vi "CRYSelect Massages.vi"(0 "Data in":T3 {"Z data" items=["dB", "Lin"]; "X data" items=["dB", "Lin"]; "Y data" items=["dB", "Lin"]; "Z dB ref" format="%.1f"; "Z axis" items=["Log", "Lin"]; "X dB ref" format="%.1f"; "X axis" items=["Log", "Lin"]; "Y axis" items=["Log", "Lin"]; "Y dB ref" format="%.1f"; "Curve"."z" format="%.2f"; "Curve"."y" format="%.2f"; "Curve"."x" format="%.2f"}, 5 "Results in":T1 {"Margin" format="%.2f"}, 7 "Mode":u16(slide), 9 "Dat_State":bool[](array[boolean]), 11 "Res_state":bool[](array[boolean]), 12 "USL":dbl, 13 "LSL":dbl) -> (4 "Run flag":bool)   [LabVIEW 2013]
uses:
  Typedef Control/CRYData Cluster Array.ctl
  Typedef Control/CRYData Cluster.ctl
  Typedef Control/CRYResult Cluster Array.ctl
  Typedef Control/CRYResult Cluster.ctl
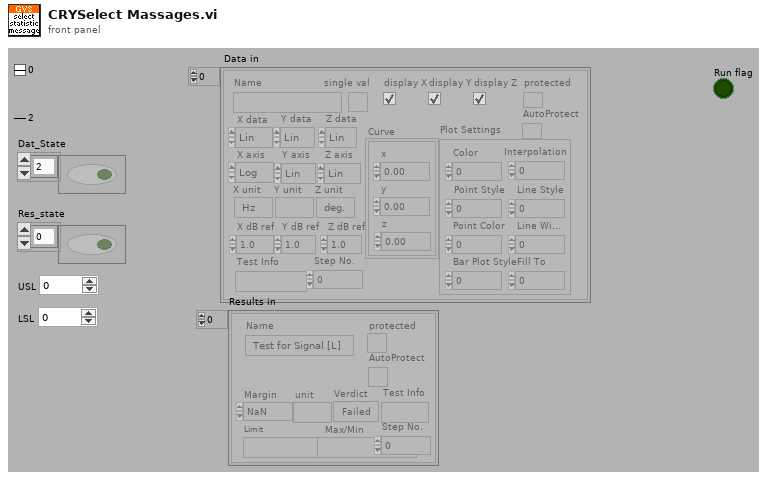
[diagram p1: front panel]
types:
  T1 = typedef "CRYResult Cluster Array.ctl" = T2[]
  T2 = typedef "CRYResult Cluster.ctl" = cluster{"Name":string, "Margin":dbl, "unit":string, "Verdict":bool, "Limit":string, "Max/Min":string, "protected":bool, "Step No.":i32, "Test Info":string, "AutoProtect":bool}
  T3 = typedef "CRYData Cluster Array.ctl" = T4[]
  T4 = typedef "CRYData Cluster.ctl" = cluster{"Name":string, "Curve":cluster{"x":dbl, "y":dbl, "z":dbl}[], "X data":u16, "Y data":u16, "Z data":u16, "X axis":u16, "Y axis":u16, "Z axis":u16, "X unit":string, "Y unit":string, "Z unit":string, "X dB ref":dbl, "Y dB ref":dbl, "Z dB ref":dbl, "single val":bool, "protected":bool, "display X":bool, "display Y":bool, "display Z":bool, "Test Info":string, "Step No.":i32, "Plot Settings":cluster{"Color":u32, "Interpolation":u8, "Point Style":u8, "Line Style":u8, "Point Color":u32, "Line Width":u8, "Bar Plot Style":u8, "Fill To":i16}, "AutoProtect":bool}
  T5 = enum16{"OK", "Yes", "YesNo", "YesNoCancel", "ReplaceAppend"}
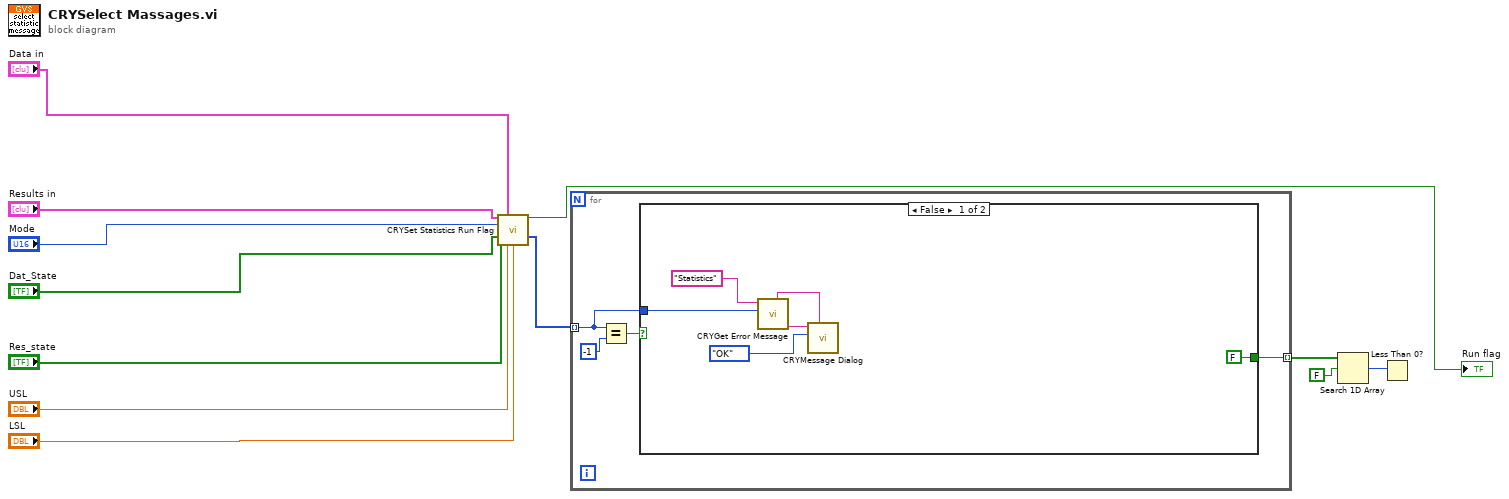
[diagram p0: block diagram]
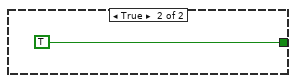
[diagram p2: hidden frame]
diagram:
  n1 = call "CRYSet Statistics Run Flag.vi"("Results in"="Results in", "Data in"="Data in", "Mode"="Mode", "Dat_State"="Dat_State", "Res_state"="Res_state", "USL"="USL", "LSL"="LSL") -> ("Run flag"=→"Run flag":bool, "Message Numbers"=w3:i32[])  [unwired: 7 in]
  n2 = for {
    tunnel: w3 -> [w13] mode=indexing
    tunnel: [w14] -> w2 mode=indexing
    n3 = Equal?(x=w13, y=-1) -> (x = y?=w15:bool)
    n4 = case shown="False" w15 {
      tunnel: [FALSE TRUE] -> w14
      tunnel: w13 -> [w19 _]
      frame False {
        n5 = call "CRYGet Error Message.vi"("Error No"=w19, "Kind"="Statistics") -> ("Message Sub 3"=w22:string, "Window Title"=w21:string)  [unwired: 4 in, 4 out]
        n6 = call "CRYMessage Dialog.vi"("Window Title"=w21, "YesNoCancel"=T5."OK", "Message Content"=w22) -> ()  [unwired: 7 in, 2 out]
      }
      frame True {
      }
    }
  }
  n7 = Search 1D Array(1D array=w2, element=FALSE) -> (index of element=w11:i32)  [unwired: 1 in]
  n8 = Less Than 0?(x=w11) -> ()  [unwired: 1 out]
